vi "bool_to_BSON_bytes.vi"(11 "value":bool) -> (3 "BSONbytes":u8[](array[numeric]))   [LabVIEW 2015, in "BSON_convertors_Library.lvlib"]
uses:
  BSON_convertors_Library.lvlib
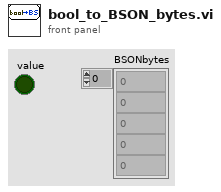
[diagram p1: front panel]
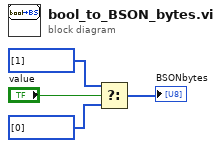
[diagram p0: block diagram]
diagram:
  n1 = Select(t=u8[] [1] ("BSONbytes"), s="value", f=u8[] [0] ("BSONbytes")) -> (s? t:f=→"BSONbytes":u8[])
